vi "TestCollectionByRef.vi"() -> ()   [LabVIEW 2021, in "Collection.lvlib"]
uses:
  Collection.lvlib
  Class 1/Class 1.lvclass
  Class 2/Class 2.lvclass
  Class 1/SetNumeric.vi
  CollectionByRef/CollectionByRef.lvclass
panel:
  out "ClassName 2":string
  out "ClassName 1":string
  out "error out":errorcluster
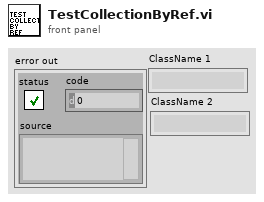
[diagram p1: front panel]
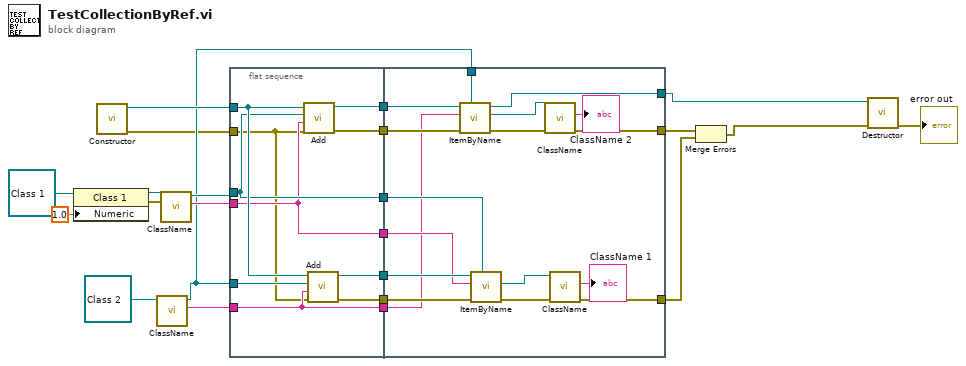
[diagram p0: block diagram]
diagram:
  n1 = property class="Class 1"(reference=refnum<class "Class 1.lvclass"> refnum ("Class 1"), "Numeric"=1.0) -> (reference out=w15:refnum<class "Class 1.lvclass">, error out=w14:errorcluster)  [unwired: 1 in]
  n2 = call "Constructor.vi"() -> ("error out"=w1:errorcluster, "CollectionByRef out"=w21:refnum<class "CollectionByRef.lvclass">)  [unwired: 10 in]
  n3 = call-dynamic "ClassName.vi"("Class 2 in"=refnum<class "Class 2.lvclass"> refnum ("Class 2")) -> ("ClassName"=w8:string, "Class 2 out"=w9:refnum<class "Class 2.lvclass">)  [unwired: 8 in, 1 out]
  n4 = call-dynamic "ClassName.vi"("error in (no error)"=w14, "Class 1 in"=w15) -> ("ClassName"=w13:string, "Class 1 out"=w12:refnum<class "Class 1.lvclass">)  [unwired: 7 in, 1 out]
  n5 = flat-sequence {
    tunnel: w12 -> [w27]
    tunnel: w21 -> [w33]
    tunnel: w9 -> [w32]
    tunnel: [w31] -> w20
    tunnel: [w30] -> w19
    tunnel: [w29] -> w18
    tunnel: [w28] -> w17
    tunnel: [w27] -> w16
    tunnel: w13 -> [w26]
    tunnel: [w26] -> w11
    tunnel: w8 -> [w25]
    tunnel: [w25] -> w7
    tunnel: w1 -> [w24]
    tunnel: w20 -> [w50]
    tunnel: w19 -> [w49]
    tunnel: w9 -> [w48]
    tunnel: w18 -> [w47]
    tunnel: w17 -> [w46]
    tunnel: w16 -> [w45]
    tunnel: w11 -> [w44]
    tunnel: w7 -> [w43]
    tunnel: [w40] -> w6
    tunnel: [w39] -> w5
    tunnel: [w37] -> w3
    frame #0 {
      n6 = call "Add.vi"("error in (no error)"=w24, "Name"=w26, "LabVIEW Object"=w27, "CollectionByRef in"=w33) -> ("error out"=w30:errorcluster, "CollectionByRef out"=w31:refnum<class "CollectionByRef.lvclass">)  [unwired: 6 in]
      n7 = call "Add.vi"("error in (no error)"=w24, "Name"=w25, "LabVIEW Object"=w32, "CollectionByRef in"=w33) -> ("error out"=w28:errorcluster, "CollectionByRef out"=w29:refnum<class "CollectionByRef.lvclass">)  [unwired: 6 in]
    }
    frame #1 {
      n8 = call "ItemByName.vi"("LabVIEW Object Type"=w48, "error in (no error)"=w49, "Name"=w43, "CollectionByRef in"=w50) -> ("error out"=w41:errorcluster, "LabVIEW Object"=w42:refnum<class "Class 2.lvclass">, "CollectionByRef out"=w40:refnum<class "CollectionByRef.lvclass">)  [unwired: 4 in, 1 out]
      n9 = call "ItemByName.vi"("LabVIEW Object Type"=w45, "error in (no error)"=w46, "Name"=w44, "CollectionByRef in"=w47) -> ("error out"=w38:errorcluster, "LabVIEW Object"=w36:refnum<class "Class 1.lvclass">)  [unwired: 4 in, 2 out]
      n10 = call-dynamic "ClassName.vi"("error in (no error)"=w41, "Class 2 in"=w42) -> ("error out"=w39:errorcluster, "ClassName"=→"ClassName 2":string)  [unwired: 7 in, 1 out]
      n11 = call-dynamic "ClassName.vi"("error in (no error)"=w38, "Class 1 in"=w36) -> ("error out"=w37:errorcluster, "ClassName"=→"ClassName 1":string)  [unwired: 7 in, 1 out]
    }
  }
  n12 = Merge Errors(w5, w3) -> (w4:errorcluster)
  n13 = call "Destructor.vi"("error in (no error)"=w4, "CollectionByRef in"=w6) -> ("error out"=→"error out":errorcluster)  [unwired: 9 in]
